vi "Timer - 1.vi"(8 "error in (no error)":errorcluster, 11 "cmd":T1) -> (0 "error out":errorcluster, 2 "update":dbl, 3 "Numeric":dbl format="%<%H:%M:%S>t")   [LabVIEW 2019]
uses:
  cmd_timer.ctl
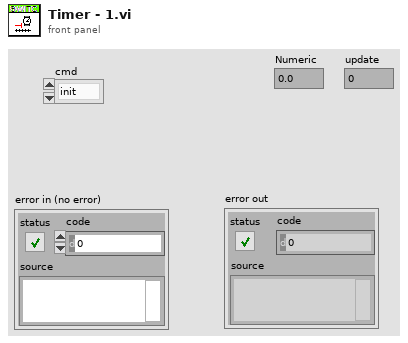
[diagram p1: front panel]
types:
  T1 = typedef "cmd_timer.ctl" = enum16{"init", "init_update", "run", "default", "update"}
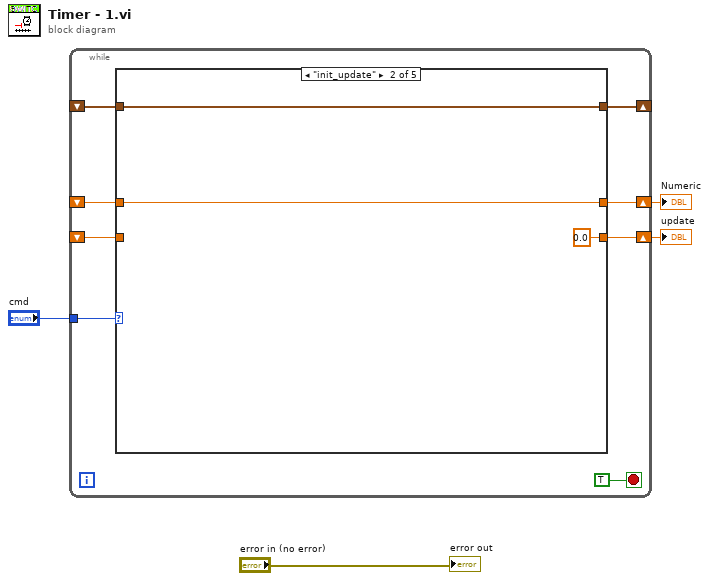
[diagram p0: block diagram]
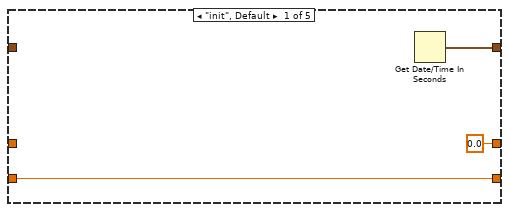
[diagram p2: hidden frame]
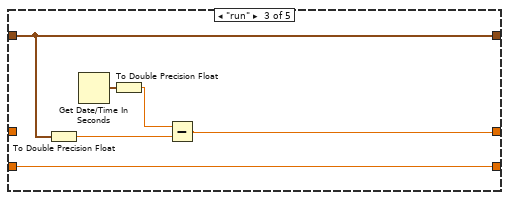
[diagram p3: hidden frame]
diagram:
  n1 = while {
    tunnel: "cmd" -> [w11]
    shift-right: [w10] -> _
    shift-left: _ -> [w9]
    shift-right: [w8] -> w2
    shift-left: _ -> [w7]
    shift-right: [w6] -> w1
    shift-left: _ -> [w5]
    stop <- TRUE stop-if-true
    n2 = case shown="\"init_update\"" w11 {
      tunnel: [w15 w18 w22 w27 w29] -> w10
      tunnel: w9 -> [_ w18 w22 w27 w29]
      tunnel: [0.0 w17 w20 w26 w28] -> w8
      tunnel: w7 -> [_ w17 _ w26 w28]
      tunnel: [w13 0.0 w19 w25 w28] -> w6
      tunnel: w5 -> [w13 _ w19 w25 _]
      frame "init", Default {
        n3 = Get Date/Time In Seconds() -> (seconds since 1Jan1904=w15:timestamp)
      }
      frame "init_update" {
      }
      frame "run" {
        n4 = To Double Precision Float(number=w22) -> (double precision float=w21:dbl)
        n5 = Get Date/Time In Seconds() -> (seconds since 1Jan1904=w23:timestamp)
        n6 = To Double Precision Float(number=w23) -> (double precision float=w24:dbl)
        n7 = Subtract(x=w24, y=w21) -> (x-y=w20:dbl)
      }
      frame "default" {
      }
      frame "update" {
      }
    }
  }
  "Numeric" <- w2
  "update" <- w1
  "error out" <- "error in (no error)"
